vi "SampleHandler.vi"() -> ()   [LabVIEW 2017]
uses:
  controls/SampleHandler_message.ctl
  controls/Stop.ctl
  controls/SampleHandler_configuration.ctl
panel:
  in  "config":T1={"port"="", "BG 1"=-82132, "BG 2"=-22571, "Sensor"=-74765, "AF 1"=-51160, "AF 2"=-123198, "AF coil"=110030, "Home (absolute)"=72, "Home (relative to limit switch)"=989}
  out "VP response":string
  out "error out":errorcluster caption="エラー出力"
  in  "error in (no error)":errorcluster caption="エラー入力（エラーなし）"
  in  "message":T2
  in  "VISAリソース名":refnum<visa-resource-name>
  # "Count (Positive=RH)"
  # "Relative to Home?"
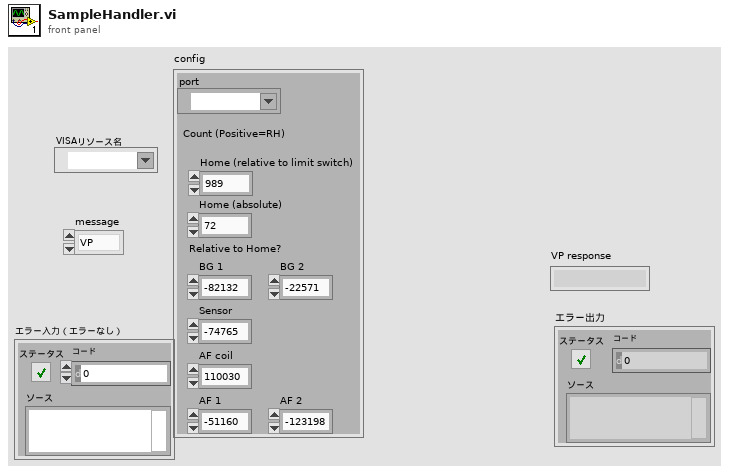
[diagram p1: front panel]
types:
  T1 = typedef "SampleHandler_configuration.ctl" = cluster{"port":refnum<visa-resource-name>, "BG 1":i32, "BG 2":i32, "Sensor":i32, "AF 1":i32, "AF 2":i32, "AF coil":i32, "Home (absolute)":i32, "Home (relative to limit switch)":i32}
  T2 = typedef "SampleHandler_message.ctl" = enum16{"VP", "home", "AF 1", "AF 2", "BG 1", "BG 2", "Sensor"}
  T3 = typedef "Stop.ctl" = enum16{"G (移動中）", "1", "2", "3", "4", "正常停止", "6", "リミットスイッチ"}
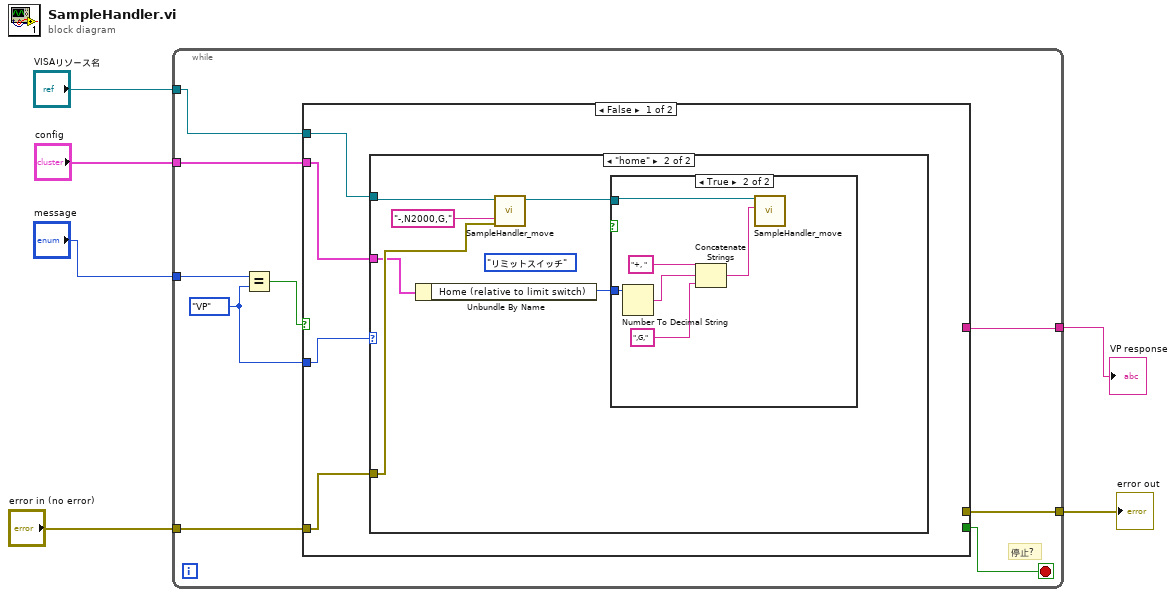
[diagram p0: block diagram]
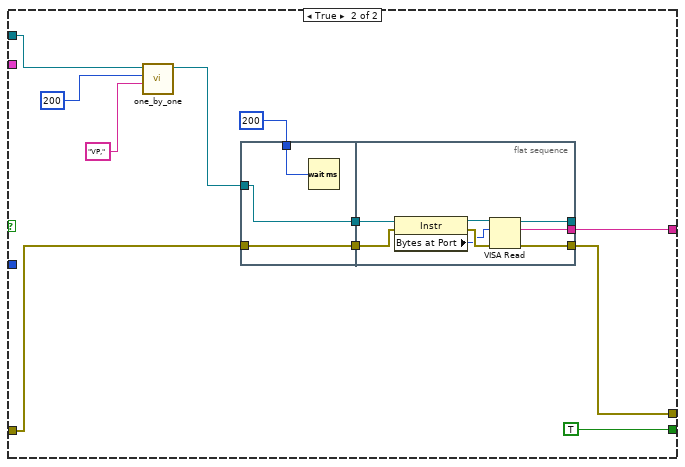
[diagram p4: hidden frame]
diagram:
  n1 = while {
    tunnel: "message" -> [w15]
    tunnel: "VISAリソース名" -> [w12]
    tunnel: "error in (no error)" -> [w11]
    tunnel: [w10] -> w3
    tunnel: [w9] -> w2
    tunnel: "config" -> [w7]
    stop <- w13 stop-if-true
    w8 = SampleHandler_message."VP" ("列挙体")
    # "停止?"
    n2 = Equal?(x=w15, y=w8) -> (x = y?=w14:bool)
    n3 = case shown="FALSE" w14 {
      tunnel: [_ TRUE] -> w13
      tunnel: w12 -> [w18 w41]
      tunnel: w11 -> [w17 w34]
      tunnel: [_ w33] -> w10
      tunnel: [_ w32] -> w9
      tunnel: w8 -> [w19 _]
      tunnel: w7 -> [w16 _]
      frame False {
        n4 = case shown="\"home\"" w19 {
          tunnel: w18 -> [_ w25]
          tunnel: w17 -> [_ w24]
          tunnel: w16 -> [_ w23]
          frame "VP", Default {
          }
          frame "home" {
            (unwired) Stop."リミットスイッチ" ("列挙体")
            n5 = Unbundle By Name(w23) -> ("Home (relative to limit switch)"=w21:i32)
            n6 = call "SampleHandler_move.vi"("error in (no error)"=w24, "移動コマンド"="-,N2000,G,", "VISAリソース名"=w25) -> ("VISAリソース名出力"=w20:refnum<visa-resource-name>)  [unwired: 6 in, 2 out]
            n7 = case shown="TRUE" {
              selector: _ -> [_ _]
              tunnel: w21 -> [_ w30]
              tunnel: w20 -> [_ w27]
              frame False {
              }
              frame True {
                n8 = Number To Decimal String(number=w30) -> (decimal integer string=w29:string)  [unwired: 1 in]
                n9 = Concatenate Strings("+, ", w29, ",G,") -> (w26:string)
                n10 = call "SampleHandler_move.vi"("移動コマンド"=w26, "VISAリソース名"=w27) -> ()  [unwired: 7 in, 3 out]
              }
            }
          }
        }
      }
      frame True {
        n11 = call "one_by_one.vi"("入力文字"="VP,", "待機 (200ms)"=200, "VISAリソース名"=w41) -> ("VISAリソース名出力"=w35:refnum<visa-resource-name>)  [unwired: 7 in, 1 out]
        n12 = flat-sequence {
          tunnel: w34 -> [w45]
          tunnel: [w43] -> w38
          tunnel: [w45] -> w37
          tunnel: i16 200 ("読み取り前待機 (500 ms)") -> [w44]
          tunnel: w35 -> [w43]
          tunnel: [w48] -> w33
          tunnel: [w47] -> _
          tunnel: [w46] -> w32
          tunnel: w38 -> [w53]
          tunnel: w37 -> [w52]
          frame #0 {
            n13 = Wait (ms)(milliseconds to wait=w44) -> ()  [unwired: 1 out]
          }
          frame #1 {
            n14 = property class="Instr"(reference=w53, error in=w52) -> (reference out=w51:refnum<visa-resource-name>, error out=w50:errorcluster, "Bytes at Port"=w49:u32)
            n15 = VISA Read(VISA resource name=w51, byte count=w49, error in (no error)=w50) -> (VISA resource name out=w47:refnum<visa-resource-name>, read buffer=w46:string, error out=w48:errorcluster)  [unwired: 1 out]
          }
        }
      }
    }
  }
  "error out" <- w3
  "VP response" <- w2
